vi "oscilloscope.vi"() -> ()   [LabVIEW 2016]
doc: "This VI illustrates how to acquire sound samples continuously from a specified device. It requires the use of a microphone attached to the sound card. You can specify the number of samples to acquire, sample rate, number of channels and a bit rate per sample. The VI also plots the raw data as the acquisition is made."
uses:
  <vilib>/sound2/lvsound2.llb/Sampling Mode.ctl
  <vilib>/measure/NI_MAPro.lvlib
  <vilib>/measure/mamon.llb/Trigger Detection for 1 Channel.vi
  flag_array.vi
  <vilib>/platform/TimedLoop/XDataNode/XDataNode.xnode
  <vilib>/Platform/TimedLoop/XDataNode/nitl_modes.ctl
  <vilib>/Platform/TimedLoop/XDataNode/XDNodeRunTimeDep.lvlib
  <vilib>/Platform/TimedLoop/XDataNode/wakeup.ctl
  <vilib>/Platform/TimedLoop/XDataNode/timing_clust.ctl
  <vilib>/Analysis/NI_AALBase.lvlib
  <vilib>/Analysis/3filter.llb/IIR Cascade Filter with I.C. (DBL).vi
  currdisp_oscillo.vi
  <vilib>/sound2/lvsound2.llb/Sound Input Read (DBL).vi
  <vilib>/sound2/lvsound2.llb/Sound File Write (DBL).vi
  <vilib>/Waveform/WDTOps.llb/WDT Index Channel DBL.vi
  <vilib>/sound2/lvsound2.llb/Sound File Write Open.vi
panel:
  in  "Sign":bool=TRUE
  in  "close \nrecording":bool
  out "Saving":bool
  in  "record":bool
  in  "stop":bool
  in  "save trace":bool
  out "input\nloop":bool[](array[boolean])
  in  "reset":bool
  in  "Trigger Mode":T1(radio)
  in  "Scope on":bool=TRUE caption="On/Off"
  in  "On/Off":bool=TRUE
  in  "Passband\nRipple (dB)":dbl=8.0 min=1.0 max=40.0 step=1.0
  in  "f":dbl=900.0 min=0.0
  in  "f":dbl=50.0 min=0.0
  in  "Order":dbl=4.0 min=1.0 max=20.0 step=1.0
  in  "Type":dbl=1.0 min=0.0 max=3.0 step=1.0
  in  "Trig. Sensitivity":dbl min=0.0 max=5.0 step=0.0001
  in  "Slope":bool=TRUE
  out "Trig'd":bool
  in  "Trigger \nLevel":dbl(slide)=0.001044849491951627 scale=1e-05..5.0
  in  "Trigger Ch.":i32=1 min=1 max=4 step=1
  out "graph":waveform(dbl)[](graph)
  in  "Bits per Sample":i32=24 min=8 max=24 step=8
  in  "Sample Rate (S/s)":dbl=44100.0
  in  "# Channels":i32=2 min=1 max=2
  in  "Device ID":u32 format="%.0x"
  in  "# Samples/Ch":i32=10000
  # "Oscilloscope"
  # "-"
  # "+"
  # "Trigger\nSensitivity"
  # "-"
  # "+"
  # "Input Filter"
  # "low"
  # "Hz"
  # "0 = Lowpass\n1 = Highpass\n2 = Bandpass\n3 = Bandstop."
  # "high"
  # "Hz"
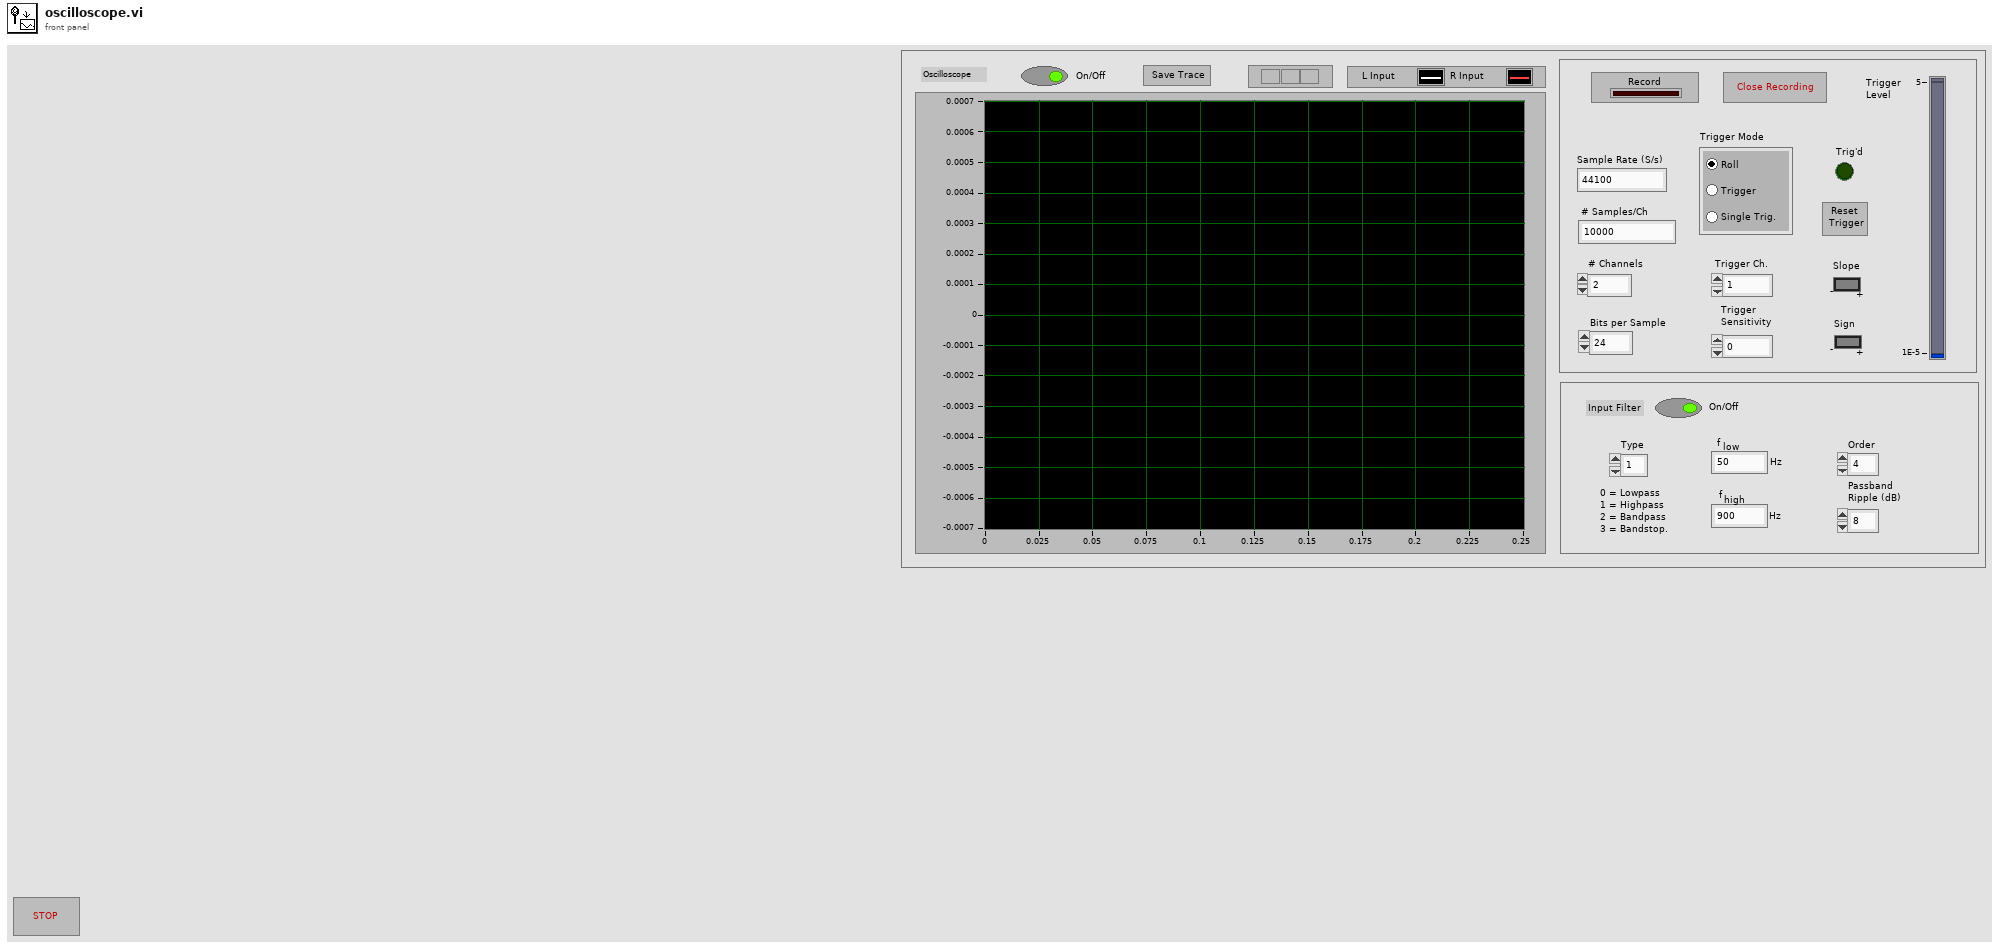
[diagram p1: front panel]
types:
  T1 = enum32{"Radio Selection 1", "Radio Selection 2", "Radio Selection 3"}
  T2 = typedef "XDNodeRunTimeDep.lvlib/timing_clust.ctl" = cluster{"Expected End [f-1]":u64, "Actual End [f-1]":u64, "Finished Late? [f-1]":bool, "Expected End [i-1]":u64, "Actual End [i-1]":u64, "Finished Late? [i-1]":bool, "Expected Start [i]":u64, "Actual Start [i]":u64, "Expected Start [f]":u64, "Actual Start [f]":u64, "Source Name":string, "Structure Name":string, "Period":i64, "Deadline":i64, "Offset":i64, "Start":i64, "Priority":i32, "Timeout":i32, "Mode":T3, "Wakeup Reason":T4, "Error":errorcluster, "Source Type":string, "Secondary Source Type":string, "Global End Time":u64, "Global Start Time":u64, "Frame Duration":u64, "Iteration Duration":u64, "Assigned CPU":i32, "I/O Scan Engine Mode":u32}
  T3 = typedef "XDNodeRunTimeDep.lvlib/nitl_modes.ctl" = enum32{"No Change", "Process missed periods, maintain original phase", "Discard missed periods, maintain original phase", "Process missed periods, ignore original phase", "Discard missed periods, ignore original phase"}
  T4 = typedef "XDNodeRunTimeDep.lvlib/wakeup.ctl" = enum32{"Normal", "Aborted", "Asynchronous wakeup", "Timing source error", "Timed loop error", "Timeout"}
  T5 = typedef "Sampling Mode.ctl" = i32
  T6 = cluster{"Sample Rate (S/s)":dbl, "# Channels":i32, "Bits per Sample":i32}
  T7 = typedef "Sound File Refnum.ctl" = refnum<file>
  T8 = typedef "Sound Input Task ID.ctl" = u32
  T9 = cluster{"filter structure":enum32{"IIR 2nd Order", "IIR 4th Order"}, "Reverse Coefficients":dbl[], "Forward Coefficients":dbl[]}
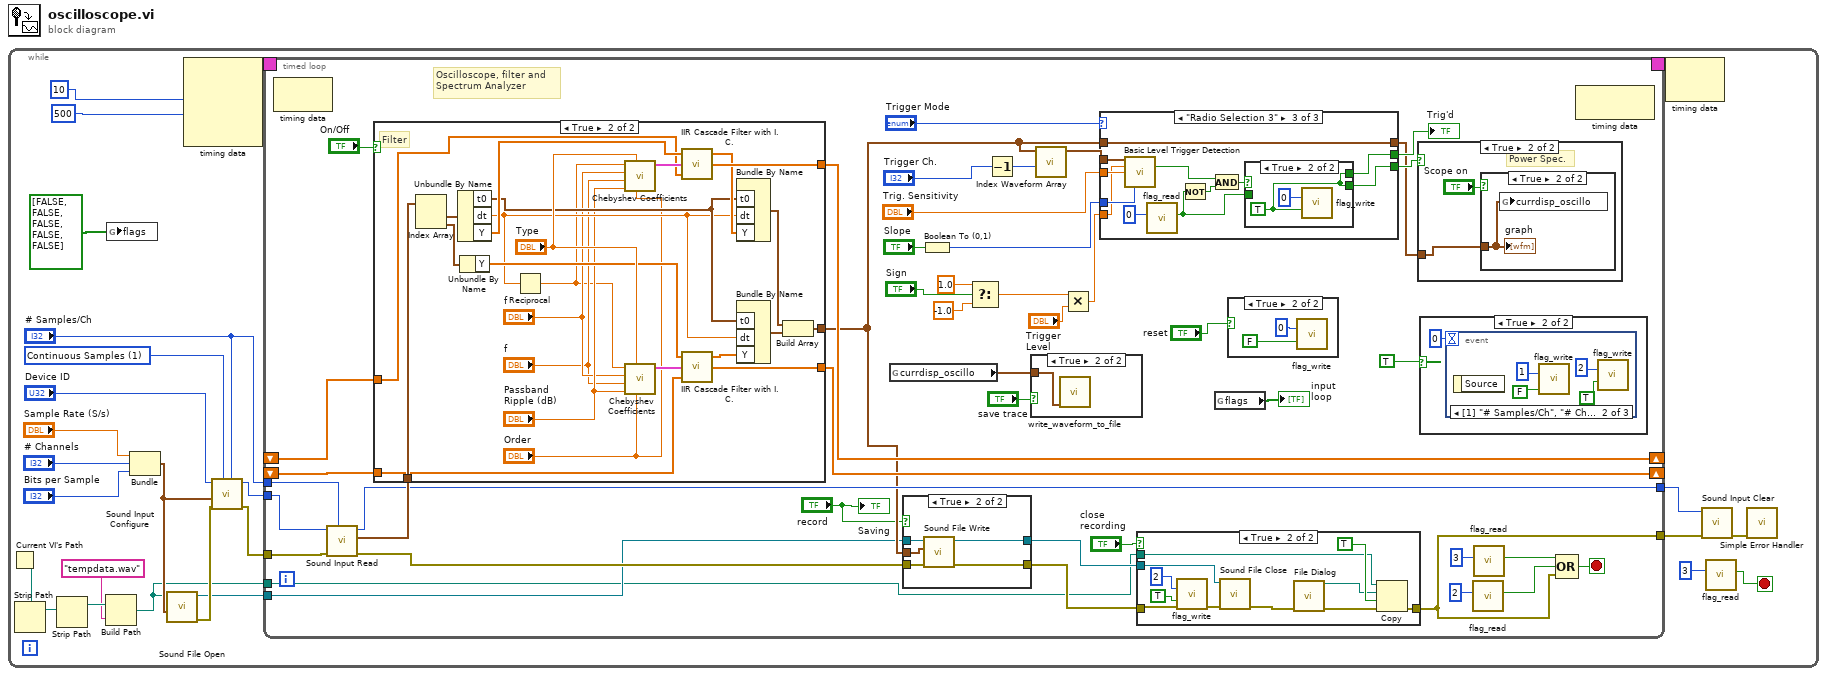
[diagram p0: block diagram]
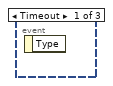
[diagram p7: hidden frame]
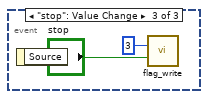
[diagram p8: hidden frame]
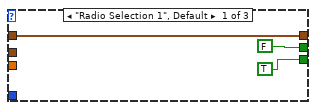
[diagram p12: hidden frame]
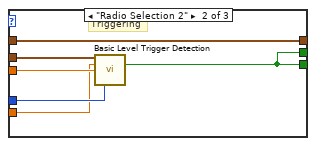
[diagram p13: hidden frame]
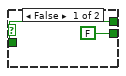
[diagram p14: hidden frame]
diagram:
  n1 = while {
    stop <- w20 stop-if-true
    w12 = T5 1 items=["Finite Samples", "Continuous Samples"] ("sample mode")
    n2 = Current VI's Path() -> (path=w6:path)
    n3 = Strip Path(path=w6) -> (stripped path=w7:path)  [unwired: 1 out]
    n4 = Strip Path(path=w7) -> (stripped path=w8:path)  [unwired: 1 out]
    n5 = Build Path(base path=w8, name or relative path="tempdata.wav") -> (appended path=w2:path)
    n6 = global write "flag_array.vi" "flags"(bool[] [FALSE, FALSE, FALSE, FALSE, FALSE]) -> ()
    n7 = Bundle("Sample Rate (S/s)"="Sample Rate (S/s)", "# Channels"="# Channels", "Bits per Sample"="Bits per Sample") -> (w3:T6)  [unwired: 1 out]
    n8 = call-poly <vilib>:"Sound File Open.vi"("sound format"=w3, "path"=w2) -> ("error out"=w4:errorcluster, "sound file refnum"=w1:T7)  [unwired: 1 in, 7 out]
    n9 = node-c288(10, 500) -> (w18:T2)  [unwired: 2 out]
    n10 = call <vilib>:"Sound Input Configure.vi"("number of samples/ch"="# Samples/Ch", "sample mode"=w12, "error in (no error)"=w4, "sound format"=w3, "device ID"="Device ID") -> ("error out"=w11:errorcluster, "task ID"=w10:T8)  [unwired: 2 in, 3 out]
    n11 = timed-loop {
      tunnel: [w52] -> w23
      tunnel: "# Samples/Ch" -> [w50]
      tunnel: [w32] -> w22
      timing: w18 -> [_]
      timing-out: [_] -> w17
      shift-right: [w56] -> _
      shift-left: _ -> [w55]
      shift-right: [w54] -> _
      shift-left: _ -> [w53]
      tunnel: w11 -> [w51]
      tunnel: w10 -> [w49]
      tunnel: w2 -> [w35]
      tunnel: w1 -> [w43]
      stop <- w33 stop-if-true
      # "Oscilloscope, filter and \nSpectrum Analyzer"
      n12 = node-c288() -> ()  [unwired: 2 out]
      n13 = call-poly <vilib>:"Sound Input Read.vi"("number of samples/ch"=w50, "error in (no error)"=w51, "task ID"=w49) -> ("error out"=w45:errorcluster, "data"=w71:waveform(dbl)[], "task ID out"=w52:T8)  [unwired: 1 in, 5 out]
      n14 = case shown="True" "On/Off" {
        tunnel: w71 -> [w103 w123]
        tunnel: [w103 w110] -> w44
        tunnel: [_ w125] -> w56
        tunnel: w55 -> [_ w124]
        tunnel: [_ w119] -> w54
        tunnel: w53 -> [_ w118]
        frame False {
        }
        frame True {
          # "Filter"
          n15 = Index Array(array=w123) -> (element #1=w117:waveform(dbl), element #2=w104:waveform(dbl))  [unwired: 2 in]
          n16 = Unbundle By Name(w117) -> ("t0"=w115:timestamp, "dt"=w114:dbl, "Y"=w126:dbl[])
          n17 = Unbundle By Name(w104) -> ("Y"=w120:dbl[])
          n18 = Reciprocal(x=w114) -> (1/x=w105:dbl)
          n19 = call <vilib>:"Chebyshev Coefficients.vi"("order"="Order", "filter type"="Type", "ripple(dB)"="Passband\nRipple (dB)", "low cutoff freq: fl"="f", "high cutoff freq: fh"="f", "sampling freq: fs"=w105) -> ("IIR Filter Cluster"=w127:T9)  [unwired: 4 in, 1 out]
          n20 = call <vilib>:"Chebyshev Coefficients.vi"("order"="Order", "filter type"="Type", "ripple(dB)"="Passband\nRipple (dB)", "low cutoff freq: fl"="f", "high cutoff freq: fh"="f", "sampling freq: fs"=w105) -> ("IIR Filter Cluster"=w121:T9)  [unwired: 4 in, 1 out]
          n21 = call-poly <vilib>:"IIR Cascade Filter with I.C..vi"("Initial Filter State"=w124, "IIR Filter Cluster"=w127, "X"=w126) -> ("Final Filter State"=w125:dbl[], "Filtered X"=w116:dbl[])  [unwired: 1 out]
          n22 = call-poly <vilib>:"IIR Cascade Filter with I.C..vi"("Initial Filter State"=w118, "IIR Filter Cluster"=w121, "X"=w120) -> ("Final Filter State"=w119:dbl[], "Filtered X"=w113:dbl[])  [unwired: 1 out]
          n23 = Bundle By Name("t0"=w115, "dt"=w114, "Y"=w116) -> (w111:waveform(dbl))  [unwired: 1 out]
          n24 = Bundle By Name("t0"=w115, "dt"=w114, "Y"=w113) -> (w112:waveform(dbl))  [unwired: 1 out]
          n25 = Build Array(w111, w112) -> (w110:waveform(dbl)[])
        }
      }
      n26 = global read "currdisp_oscillo.vi" "currdisp_oscillo"() -> (w47:waveform(dbl)[])
      n27 = case shown="True" "record" {
        tunnel: w45 -> [w73 w74]
        tunnel: [w73 w78] -> w41
        tunnel: w44 -> [_ w77]
        tunnel: w43 -> [w72 w76]
        tunnel: [w72 w75] -> w40
        frame False {
        }
        frame True {
          n28 = call-poly <vilib>:"Sound File Write.vi"("error in (no error)"=w74, "data"=w77, "sound file refnum"=w76) -> ("error out"=w78:errorcluster, "sound file refnum out"=w75:T7)  [unwired: 7 out]
        }
      }
      n29 = Boolean To (0,1)(Boolean="Slope") -> (0, 1=w63:i16)
      n30 = Select(t=1.0, s="Sign", f=-1.0) -> (s? t:f=w27:dbl)
      n31 = Decrement(x="Trigger Ch.") -> (x-1=w67:i32)
      n32 = case shown="True" "save trace" {
        tunnel: w47 -> [_ w93]
        frame False {
        }
        frame True {
          n33 = call "write_waveform_to_file.vi"("Waveform Array"=w93) -> ()  [unwired: 3 in, 8 out]
        }
      }
      n34 = call-poly <vilib>:"Index Waveform Array.vi"("index"=w67, "waveform array"=w44) -> ("waveform"=w64:waveform(dbl))  [unwired: 1 in, 8 out]
      n35 = Multiply(x=w27, y="Trigger \nLevel") -> (x*y=w37:dbl)
      n36 = case shown="\"Radio Selection 3\"" "Trigger Mode" {
        tunnel: [w131 w136 w149] -> w58
        tunnel: w44 -> [w131 w136 w149]
        tunnel: [TRUE w139 w142] -> w69
        tunnel: [FALSE w139 w141] -> w68
        tunnel: "Trig. Sensitivity" -> [_ w138 w148]
        tunnel: w64 -> [_ w137 w150]
        tunnel: w63 -> [_ w135 w151]
        tunnel: w37 -> [_ w134 w140]
        frame "Radio Selection 1", Default {
        }
        frame "Radio Selection 2" {
          # "Triggering"
          n37 = call-poly <vilib>:"Basic Level Trigger Detection.vi"("signal in"=w137, "level"=w134, "hysteresis"=w138, "trigger slope"=w135) -> ("trigger detected?"=w139:bool)  [unwired: 3 in, 8 out]
        }
        frame "Radio Selection 3" {
          n38 = call-poly <vilib>:"Basic Level Trigger Detection.vi"("signal in"=w150, "level"=w140, "hysteresis"=w148, "trigger slope"=w151) -> ("trigger detected?"=w144:bool)  [unwired: 3 in, 8 out]
          n39 = call "flag_read.vi"("flag number"=0) -> ("flag value"=w143:bool)  [unwired: 1 in, 9 out]
          n40 = Not(x=w143) -> (.not. x?=w147:bool)
          n41 = And(x=w144, y=w147) -> (x .and. y?=w146:bool)
          n42 = case shown="True" w146 {
            tunnel: [w153 w154] -> w141
            tunnel: w143 -> [w153 _]
            tunnel: [FALSE w154] -> w142
            frame False {
            }
            frame True {
              w154 = TRUE
              n43 = call "flag_write.vi"("flag number"=0, "flag value"=w154) -> ()  [unwired: 1 in, 13 out]
            }
          }
        }
      }
      "Trig'd" <- w68
      n44 = case shown="True" "close \nrecording" {
        tunnel: w40 -> [_ w88]
        tunnel: w41 -> [w79 w86]
        tunnel: w35 -> [_ w80]
        tunnel: [w79 w83] -> w32
        frame False {
        }
        frame True {
          n45 = call "flag_write.vi"("flag number"=2, "flag value"=TRUE, "error in (no error)"=w86) -> ("error out"=w87:errorcluster)  [unwired: 12 out]
          n46 = call <vilib>:"Sound File Close.vi"("error in (no error)"=w87, "sound file refnum"=w88) -> ("error out"=w84:errorcluster)  [unwired: 9 out]
          n47 = call "File Dialog"("error in"=w84) -> ("selected path"=w81:path, "error out"=w85:errorcluster)  [unwired: 6 in, 7 out]
          n48 = Copy(8:w85, 9:TRUE, 10:w81, 11:w80) -> (0:w83:errorcluster)  [unwired: 3 out]
        }
      }
      n49 = global read "flag_array.vi" "flags"() -> (→"input\nloop":bool[])
      n50 = case shown="True" "reset" {
        frame False {
        }
        frame True {
          n51 = call "flag_write.vi"("flag number"=0, "flag value"=FALSE) -> ()  [unwired: 1 in, 13 out]
        }
      }
      n52 = case shown="True" w69 {
        tunnel: w58 -> [_ w129]
        frame False {
        }
        frame True {
          # "Power Spec."
          n53 = case shown="True" "Scope on" {
            tunnel: w129 -> [_ w130]
            frame False {
            }
            frame True {
              n54 = global write "currdisp_oscillo.vi" "currdisp_oscillo"(w130) -> ()
              "graph" <- w130
            }
          }
        }
      }
      n55 = case shown="True" TRUE {
        frame False {
        }
        frame True {
          n56 = event shown="[1] \"# Samples/Ch\", \"# Channels\", \"Bits per Sample\", \"Trigger Ch.\", \"Slope\", \"Type\", \"Order\", \"f\", \"f\", \"Passband Ripple (dB)\", \"Trigger Mode\", \"Sample Rate (S/s)\": Value Change" {
            selector: _ -> [_ _ _]
            dyn-events: _ -> [_ _ _]
            timeout: 0 -> [_ _ _]
            event Timeout {
              n57 = event-data() -> ()  [unwired: 2 out]
            }
            event "# Samples/Ch", "# Channels", "Bits per Sample", "Trigger Ch.", "Slope", "Type", "Order", "f", "f", "Passband\nRipple (dB)", "Trigger Mode", "Sample Rate (S/s)": Value Change {
              n58 = event-data() -> ()  [unwired: 2 out]
              n59 = call "flag_write.vi"("flag number"=1, "flag value"=FALSE) -> ()  [unwired: 1 in, 13 out]
              n60 = call "flag_write.vi"("flag number"=2, "flag value"=TRUE) -> ()  [unwired: 1 in, 13 out]
            }
            event "stop": Value Change {
              n61 = event-data() -> ()  [unwired: 2 out]
              n62 = call "flag_write.vi"("flag number"=3, "flag value"="stop") -> ()  [unwired: 1 in, 13 out]
            }
          }
        }
      }
      n63 = call "flag_read.vi"("flag number"=2) -> ("flag value"=w34:bool)  [unwired: 1 in, 9 out]
      n64 = call "flag_read.vi"("flag number"=3) -> ("flag value"=w31:bool)  [unwired: 1 in, 9 out]
      n65 = Compound Arithmetic op=OR(w31, w34, w32) -> (w33:bool)
      n66 = node-c288() -> ()  [unwired: 2 out]
      "Saving" <- "record"
    }
    n67 = node-c288(w17) -> ()  [unwired: 1 out]
    n68 = call <vilib>:"Sound Input Clear.vi"("error in (no error)"=w22, "task ID"=w23) -> ("error out"=w9:errorcluster)  [unwired: 9 out]
    n69 = call "flag_read.vi"("flag number"=3) -> ("flag value"=w20:bool)  [unwired: 1 in, 9 out]
    n70 = call <vilib>:"Simple Error Handler.vi"("error in (no error)"=w9) -> ()  [unwired: 1 in, 8 out]
  }
